vi "Subtract Baseline.vi"(9 "Do something?":bool=TRUE, 11 "image array in":u16[][][](array[numeric])) -> (3 "image array out":u16[][][](array[numeric]))   [LabVIEW 2023]
uses:
  <vilib>/Analysis/NI_AALBase.lvlib
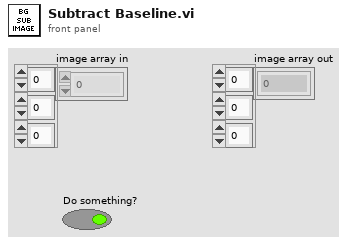
[diagram p1: front panel]
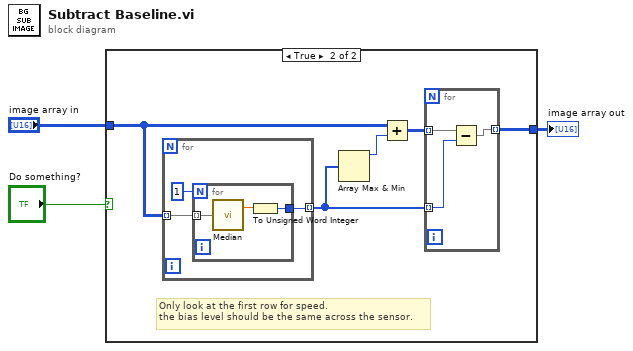
[diagram p0: block diagram]
diagram:
  n1 = case shown="True" "Do something?" {
    tunnel: "image array in" -> [w4 w8]
    tunnel: [w4 w7] -> w2
    frame False {
    }
    frame True {
      # "Only look at the first row for speed.\nthe bias level should be the same across the sensor."
      n2 = for "For each camera..." {
        tunnel: w8 -> [w11] mode=indexing
        tunnel: [w10] -> w6 mode=indexing
        # "For each camera..."
        n3 = for {
          N: 1 -> [_]
          tunnel: w11 -> [w15] mode=indexing
          tunnel: [w13] -> w10
          n4 = call <vilib>:"Median.vi"("X"=w15) -> ("median"=w14:dbl)  [unwired: 1 out]
          n5 = To Unsigned Word Integer(number=w14) -> (unsigned 16bit integer=w13:u16)
        }
      }
      n6 = Array Max & Min(array=w6) -> (max value=w5:u16)  [unwired: 3 out]
      n7 = Add(x=w8, y=w5) -> (x+y=w9:u16[][][])
      n8 = for {
        tunnel: [w16] -> w7 mode=indexing
        tunnel: w9 -> [w18] mode=indexing
        tunnel: w6 -> [w17] mode=indexing
        n9 = Subtract(x=w18, y=w17) -> (x-y=w16:u16[][])
      }
    }
  }
  "image array out" <- w2
